vi "QueueFGV.vi"(7 "Mode (get)":enum16{"set", "get"}(ring)=enum."get", 8 "error in (no error)":errorcluster, 11 "Queues":T1) -> (0 "error out":errorcluster, 3 "Queues out":T1)   [LabVIEW 2019, in "RT_Game.lvlib" / "Engine.lvclass"]
uses:
  Engine.lvclass
  Queues.ctl
  MessageCluster.ctl
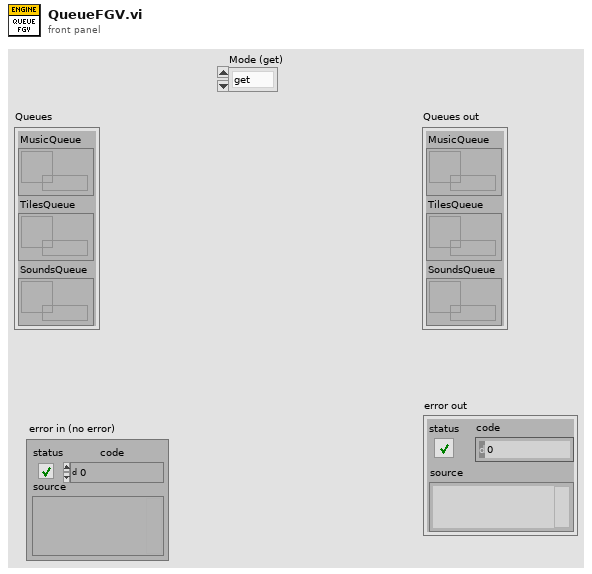
[diagram p1: front panel]
types:
  T1 = typedef "RT_Game.lvlib/Engine.lvclass/Queues.ctl" = cluster{"MusicQueue":refnum<queue>, "TilesQueue":refnum<queue>, "SoundsQueue":refnum<queue>}
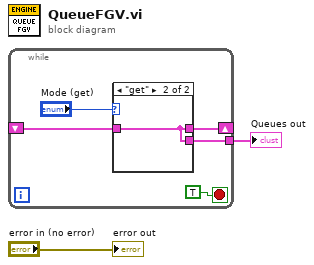
[diagram p0: block diagram]
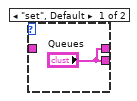
[diagram p2: hidden frame]
diagram:
  n1 = while {
    shift-right: [w6] -> _
    shift-left: _ -> [w5]
    tunnel: [w4] -> w2
    stop <- TRUE stop-if-true
    n2 = case shown="\"get\"" "Mode (get)" {
      tunnel: ["Queues" w9] -> w6
      tunnel: w5 -> [_ w9]
      tunnel: ["Queues" w9] -> w4
      frame "set", Default {
      }
      frame "get" {
      }
    }
  }
  "Queues out" <- w2
  "error out" <- "error in (no error)"
